vi "ReadWrite.ProcessData.Reset.vi"(8 "error in (no error)":errorcluster, 10 "timeout ms":i32=100, 11 "ReadWrite in":refnum<class "ReadWrite.lvclass">) -> (0 "error out":errorcluster, 1 "Timeout?":bool, 3 "ReadWrite out":refnum<class "ReadWrite.lvclass">)   [LabVIEW 2015, in "Data Access Engine.lvlib" / "ReadWrite.lvclass"]
uses:
  ReadWrite.lvclass
  ReadWrite.lvclass/ReadWrite.ctl
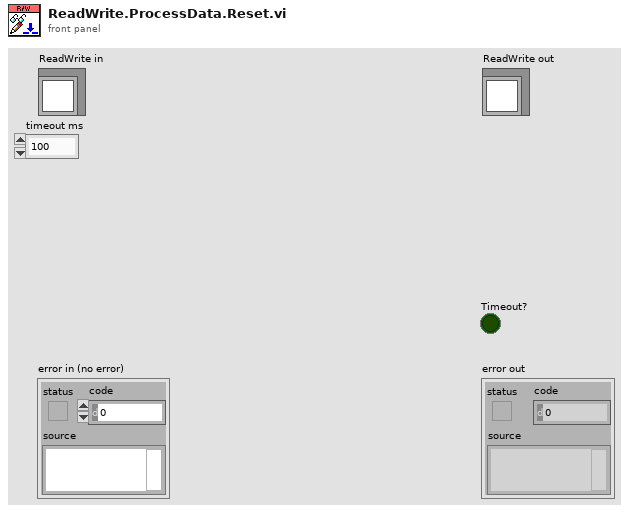
[diagram p1: front panel]
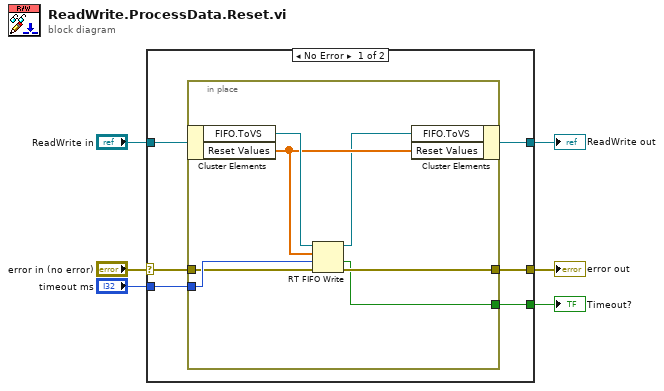
[diagram p0: block diagram]
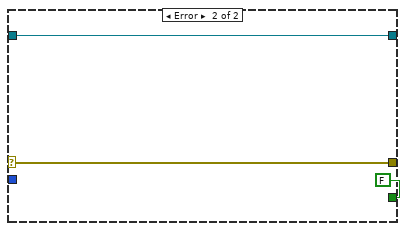
[diagram p2: hidden frame]
diagram:
  n1 = case shown="No Error" "error in (no error)" {
    selector: "error in (no error)" -> [w12 w20]
    tunnel: [w11 w20] -> w5
    tunnel: [w9 w21] -> w3
    tunnel: "ReadWrite in" -> [w10 w21]
    tunnel: "timeout ms" -> [w8 _]
    tunnel: [w7 FALSE ("empty?")] -> w1
    frame No Error {
      n2 = in-place {
        in-place-border: w12 -> [w13]
        in-place-border: [w16] -> w11
        in-place-border: w8 -> [w14]
        in-place-border: [w15] -> w7
        n3 = in-place-cluster #1(w10) -> ("FIFO.ToVS"=w19:refnum<k33>, "Reset Values"=w18:dbl[])
        n4 = RT FIFO Write(0:w19, 1:w18, 2:w14, 3:w13) -> (8:w17:refnum<k33>, 10:w15:bool, 11:w16:errorcluster)  [unwired: 1 in, 1 out]
        n5 = in-place-cluster #1("FIFO.ToVS"=w17, "Reset Values"=w18) -> (w9:refnum<class "ReadWrite.lvclass">)
      }
    }
    frame Error {
    }
  }
  "error out" <- w5
  "ReadWrite out" <- w3
  "Timeout?" <- w1
